vi "2100_Test_Set State_Measure iVIO only.vi"(0 "Semiconductor Module Context":T4, 1 "All_Scripts":string[][](array[string]), 2 "Master_Register_Data_Array_In":T1 {"Address" format="%.0x"}, 3 "Publishable IDs":string[](array[string])=["LowPower", "Active"], 4 "USID":T3 max=15, 5 "Error In":errorcluster, 7 "SMU_Pins":string[](array[string])=["VSU"], 11 "HSDIO_Pins":string[](array[string])=["CLK", "SDA"], 13 "Script Name":string="WalkingState") -> (15 "Master_Register_Data_Array_Out":T1 {"Address" format="%.0x"}, 19 "Error Out":errorcluster)   [LabVIEW 2013]
uses:
  Controls/USID.ctl
  <vilib>/NI_TestStand_SemiconductorModule/NI_TestStand_Semiconductor_Module.lvlibp/PinMap/General/SemiconductorModuleContext.ctl
  Controls/Master_Reg_Data_Array.ctl
  Controls/Reg_Address_Data.ctl
  <instrlib>/niDCPower/nidcpower.llb/niDCPower Measurement Type.ctl
  <vilib>/NI_TestStand_SemiconductorModule/NI_TestStand_Semiconductor_Module.lvlibp/PinMap/DC Power/PinsToNIDCPowerSessions.vi
  <vilib>/NI_TestStand_SemiconductorModule/NI_TestStand_Semiconductor_Module.lvlibp/PinMap/General/Publish/PublishDataDouble2D.vi
  <vilib>/NI_TestStand_SemiconductorModule/NI_TestStand_Semiconductor_Module.lvlibp
panel:
  in  "Tab Control":enum32{"Test Info", "Instrument Settings"}(tab)
  out "Current measurements":dbl[][](array[numeric])
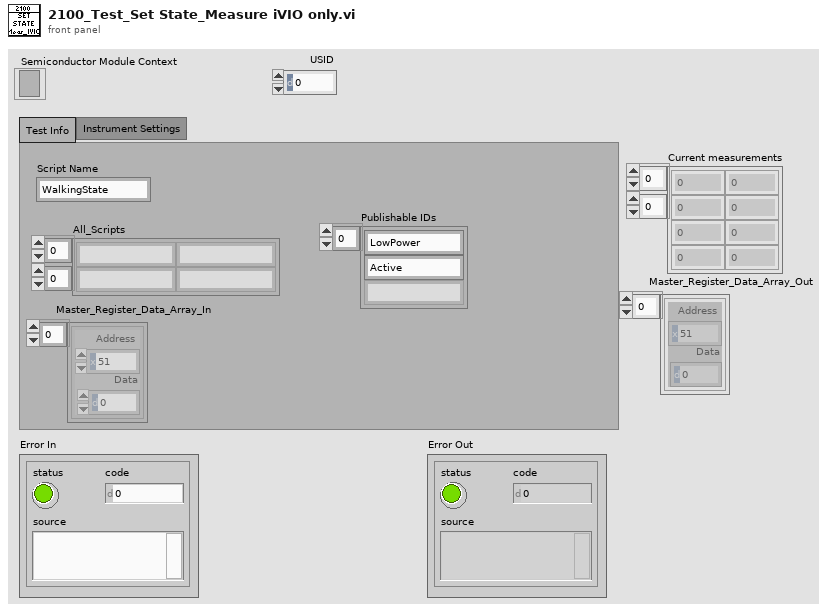
[diagram p1: front panel]
types:
  T1 = typedef "Master_Reg_Data_Array.ctl" = T2[]
  T2 = typedef "Reg_Address_Data.ctl" = cluster{"Address":u8, "Data":u8}
  T3 = typedef "USID.ctl" = u8
  T4 = typedef "NI_TestStand_Semiconductor_Module.lvlibp/SemiconductorModuleContext.ctl" = refnum<k7>
  T5 = typedef "Script Functions_Array.ctl" = enum16{"Reg_Write", "Bit_Write", "Delay", "Read"}[]
  T6 = enum16{"Reg_Write", "Bit_Write", "Delay", "Read"}
  T7 = typedef "niDCPower Measurement Type.ctl" = i32
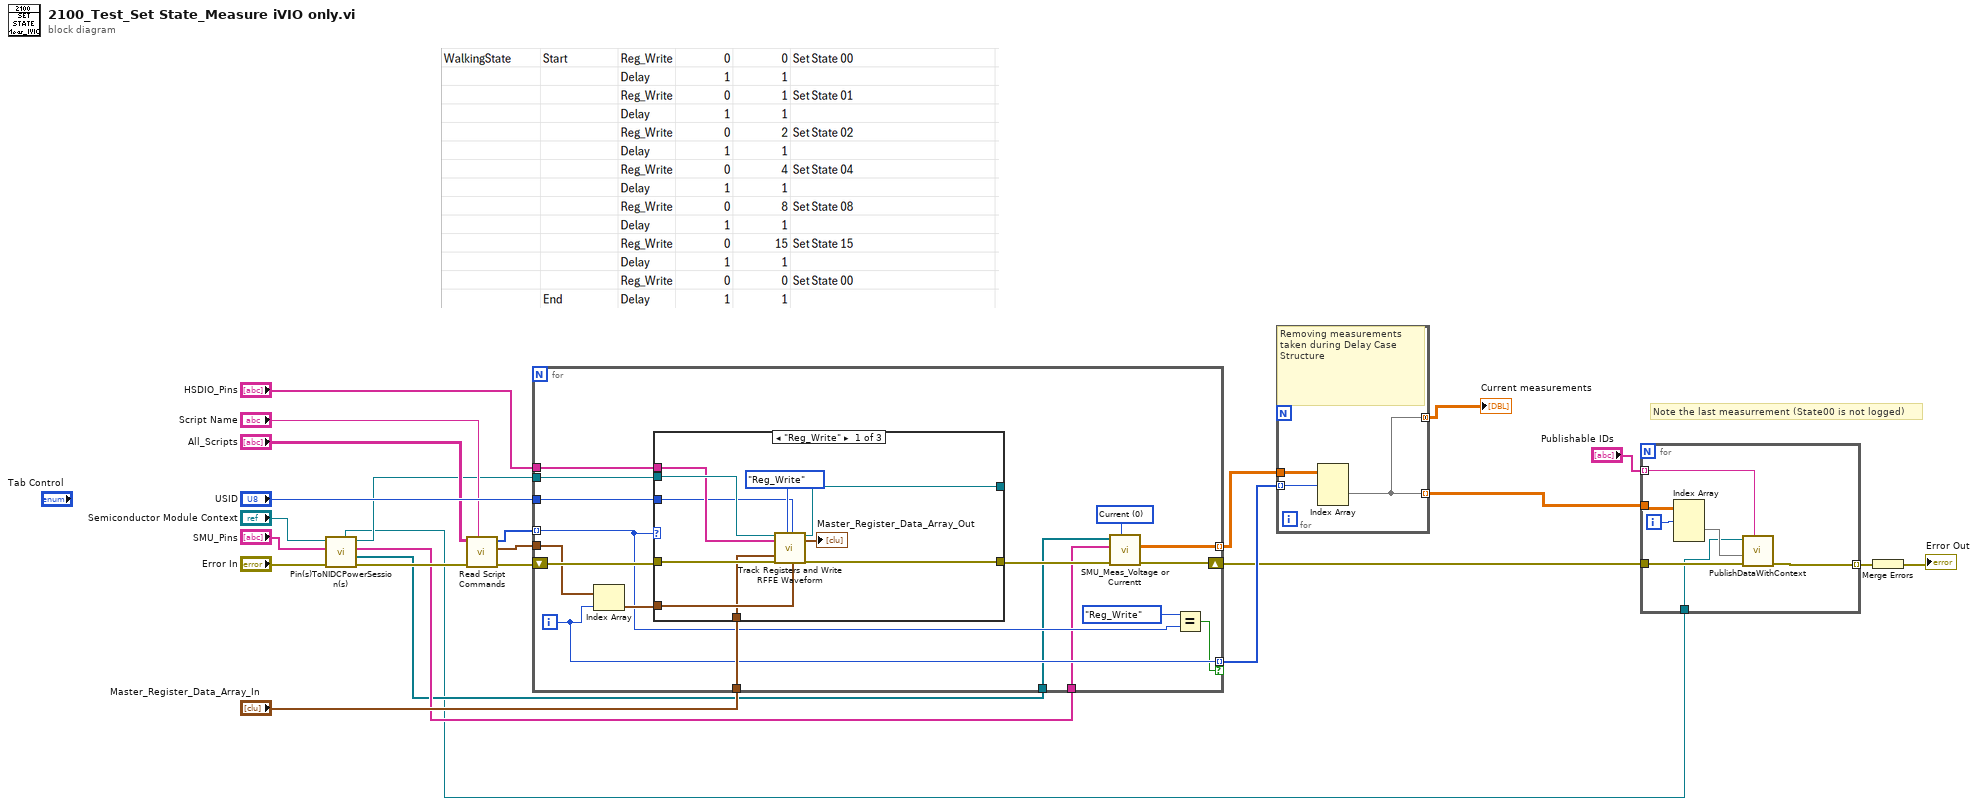
[diagram p0: block diagram]
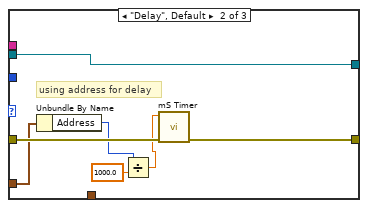
[diagram p2: hidden frame]
diagram:
  # "Note the last measurrement (State00 is not logged)"
  n1 = call-poly <vilib>:"Pin(s)ToNIDCPowerSession(s).vi"("error in (no error)"="Error In", "Pins"="SMU_Pins", "Semiconductor Module Context"="Semiconductor Module Context") -> ("error out"=w8:errorcluster, "Instrument Sessions"=w6:refnum<k15>[], "Channel Lists"=w7:string[], "Semiconductor Module Context Out"=w11:T4, "Pin Query Context"=w3:refnum<class "MultiplePinMultipleSessionQueryContext.lvclass">)  [unwired: 4 in]
  n2 = call "Read Script Commands.vi"("Test Name"="Script Name", "Error In"=w8, "All_Scripts"="All_Scripts") -> ("Error Out"=w19:errorcluster, "Script_Data"=w20:T2[], "Script_Functions"=w21:T5)  [unwired: 6 in]
  n3 = for {
    tunnel: "USID" -> [w35]
    tunnel: w21 -> [w33] mode=indexing
    tunnel: w20 -> [w38]
    tunnel: w11 -> [w40]
    tunnel: "HSDIO_Pins" -> [w39]
    shift-right: [w25] -> w13
    shift-left: w19 -> [w41]
    tunnel: "Master_Register_Data_Array_In" -> [w36]
    tunnel: [w32] -> w14 mode=indexing if=w31
    tunnel: w7 -> [w28]
    tunnel: w6 -> [w29]
    tunnel: [w26] -> w5 mode=indexing
    i -> [w32]
    w27 = T7 0 items=["Current", "Voltage"] ("measurement type")
    n4 = Index Array(array=w38, index=w32) -> (element=w37:T2)
    n5 = case shown="\"Reg_Write\"" w33 {
      tunnel: w37 -> [w45 w57 _]
      tunnel: w41 -> [w51 w58 w60]
      tunnel: w35 -> [w42 _ _]
      tunnel: w40 -> [w49 w55 w59]
      tunnel: w39 -> [w47 _ _]
      tunnel: [w50 w56 w60] -> w30
      tunnel: [w48 w55 w59] -> _
      tunnel: w36 -> [w44 _ _]
      frame "Reg_Write" {
        n6 = call "Track Registers and Write RFFE Waveform.vi"("Semiconductor Module Context"=w49, "Pins"=w47, "Master_Register_Data_Array_In"=w44, "Error In"=w51, "Script_Functions"=enum16{"Reg_Write", "Bit_Write"}."Reg_Write", "USID"=w42, "Reg_Address_Data"=w45) -> ("Semiconductor Module Context Out"=w48:T4, "Master_Register_Data_Array_Out"=→"Master_Register_Data_Array_Out":T1, "Error Out"=w50:errorcluster)  [unwired: 10 in]
      }
      frame "Delay", Default {
        # "using address for delay"
        n7 = Unbundle By Name(w57) -> ("Address"=w53:u8)
        n8 = Divide(x=w53, y=1000.0) -> (x/y=w52:dbl)
        n9 = call "mS Timer.vi"("Error In"=w58, "Delay(S)"=w52) -> ("Error Out"=w56:errorcluster)  [unwired: 9 in]
      }
      frame "Read" {
      }
    }
    n10 = call "SMU_Meas_Voltage or Currentt.vi"("measurement type"=w27, "error in (no error)"=w30, "Channel Lists"=w28, "DCPower Sessions In"=w29) -> ("error out"=w25:errorcluster, "Measurement"=w26:dbl[][])  [unwired: 5 in, 1 out]
    n11 = Equal?(x=T6."Reg_Write" ("Enum"), y=w33) -> (x = y?=w31:bool)
  }
  n12 = for {
    tunnel: w14 -> [w63] mode=indexing
    tunnel: [w61] -> w1 mode=indexing
    tunnel: w5 -> [w62]
    tunnel: [w61] -> w4 mode=concatenating
    # "Removing measurements taken during Delay Case Structure"
    n13 = Index Array(array=w62, index (dim 0)=w63) -> (element=w61:dbl[][])  [unwired: 2 in]
  }
  "Current measurements" <- w4
  n14 = for {
    tunnel: "Publishable IDs" -> [w70] mode=indexing
    tunnel: [w69] -> w15 mode=indexing
    tunnel: w13 -> [w68]
    tunnel: w1 -> [w67]
    tunnel: w3 -> [w64]
    i -> [w66]
    n15 = Index Array(array=w67, index (dim 0)=w66) -> (element=w65:dbl[][])  [unwired: 2 in]
    n16 = call-poly <vilib>:"PublishDataWithContext.vi"("Published Data Id"=w70, "error in (no error)"=w68, "Data In"=w65, "Pin Query Context"=w64) -> ("error out"=w69:errorcluster)  [unwired: 6 in, 1 out]
  }
  n17 = Merge Errors(w15) -> (→"Error Out":errorcluster)
